vi "232_fgv.vi"(7 "cmd":enum16{"close", "ini", "read", "write"}(ring), 8 "error in":errorcluster, 9 "write buffer":string, 10 "baud rate (9600)":u32=9600, 11 "VISA resource name":refnum<visa-resource-name>) -> (0 "error out":errorcluster, 3 "read buffer":string)   [LabVIEW 2018]
uses:
  <vilib>/Instr/_visa.llb/VISA Configure Serial Port (Instr).vi
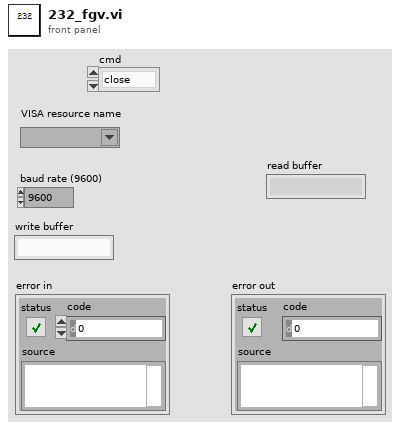
[diagram p1: front panel]
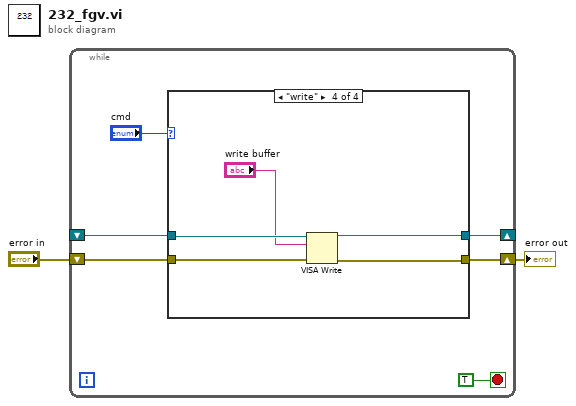
[diagram p0: block diagram]
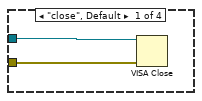
[diagram p2: hidden frame]
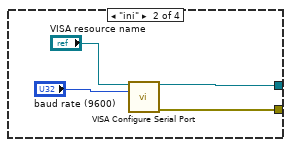
[diagram p3: hidden frame]
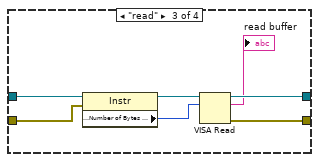
[diagram p4: hidden frame]
diagram:
  n1 = while {
    shift-right: [w5] -> w2
    shift-left: "error in" -> [w4]
    shift-right: [w6] -> _
    shift-left: _ -> [w3]
    stop <- TRUE stop-if-true
    n2 = case shown="\"write\"" "cmd" {
      tunnel: [_ w12 w17 w24] -> w6
      tunnel: [_ w11 w16 w25] -> w5
      tunnel: w4 -> [w10 _ w21 w26]
      tunnel: w3 -> [w9 _ w20 w23]
      frame "close", Default {
        n3 = VISA Close(VISA resource name=w9, error in (no error)=w10) -> ()  [unwired: 1 out]
      }
      frame "ini" {
        n4 = call-poly "VISA Configure Serial Port"("VISA resource name"="VISA resource name", "baud rate (9600)"="baud rate (9600)") -> ("VISA resource name out"=w12:refnum<visa-resource-name>, "error out"=w11:errorcluster)  [unwired: 12 in]
      }
      frame "read" {
        n5 = property class="Instr"(reference=w20, error in=w21) -> (reference out=w18:refnum<visa-resource-name>, "Serial Settings:Number of Bytes at Serial Port"=w19:u32)  [unwired: 1 out]
        n6 = VISA Read(VISA resource name=w18, byte count=w19) -> (VISA resource name out=w17:refnum<visa-resource-name>, read buffer=→"read buffer":string, error out=w16:errorcluster)  [unwired: 1 in, 1 out]
      }
      frame "write" {
        n7 = VISA Write(VISA resource name=w23, write buffer="write buffer", error in (no error)=w26) -> (VISA resource name out=w24:refnum<visa-resource-name>, error out=w25:errorcluster)  [unwired: 1 out]
      }
    }
  }
  "error out" <- w2
